vi "SaveProject.vi"(8 "error in (no error)":errorcluster, 9 "Path":path, 10 "BrowerComponent":refnum<class "BrowerComponent.lvclass">, 11 "FileController in":refnum<class "ProjectController.lvclass">) -> (0 "error out":errorcluster, 3 "FileController out":refnum<class "ProjectController.lvclass">)   [LabVIEW 2015, in "ProjectController.lvclass"]
uses:
  ProjectController.lvclass
  Brower Console/Models/BrowerComponent/BrowerComponent/BrowerComponent.lvclass
  ProjectController.lvclass/ProjectController.ctl
  Models/ProjectManager/XML Project.lvclass
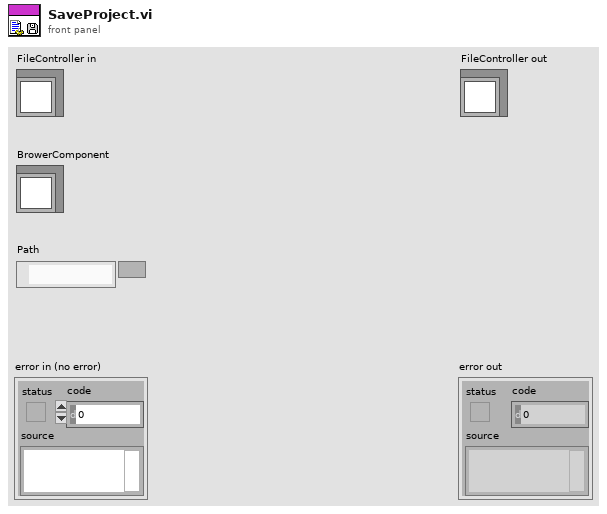
[diagram p1: front panel]
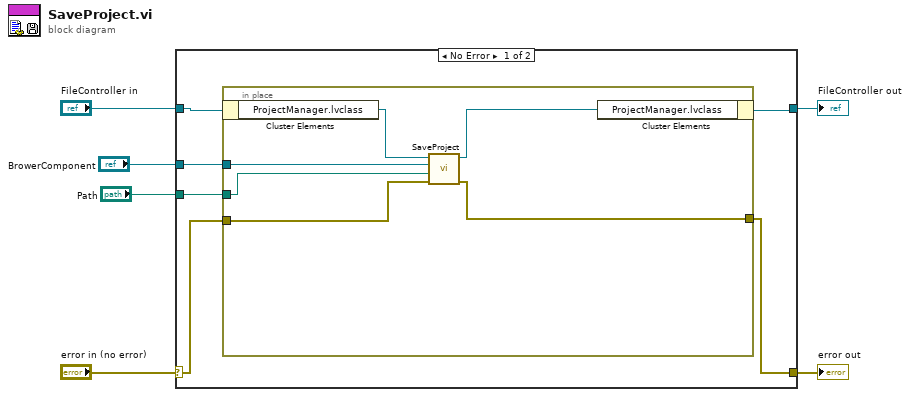
[diagram p0: block diagram]
diagram:
  n1 = case shown="No Error" "error in (no error)" {
    selector: "error in (no error)" -> [w9 w20]
    tunnel: [w8 w20] -> w5
    tunnel: [w7 w19] -> w3
    tunnel: "FileController in" -> [w12 w19]
    tunnel: "BrowerComponent" -> [w11 _]
    tunnel: "Path" -> [w10 _]
    frame No Error {
      n2 = in-place {
        in-place-border: w11 -> [w17]
        in-place-border: w10 -> [w16]
        in-place-border: w9 -> [w15]
        in-place-border: [w13] -> w8
        n3 = in-place-cluster #1(w12) -> ("ProjectManager.lvclass"=w18:refnum<class "XML Project.lvclass">)
        n4 = call "SaveProject.vi"("error in (no error)"=w15, "XML File Path"=w16, "BrowerComponent"=w17, "XML Project"=w18) -> ("error out"=w13:errorcluster, "ProjectManager out"=w14:refnum<class "XML Project.lvclass">)  [unwired: 6 in]
        n5 = in-place-cluster #1("ProjectManager.lvclass"=w14) -> (w7:refnum<class "ProjectController.lvclass">)
      }
    }
    frame Error {
    }
  }
  "error out" <- w5
  "FileController out" <- w3
